vi "WinCI Convert Adv Options.vi"(4 "advanced options":variant) -> (1 "command options":u32)   [LabVIEW 2020, in "NI_SCC_WinCI.lvlib"]
uses:
  <vilib>/SourceControl/Providers/WinCI/NI_SCC_WinCI.lvlib
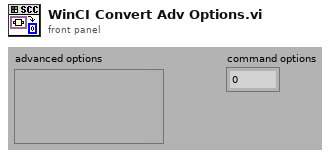
[diagram p1: front panel]
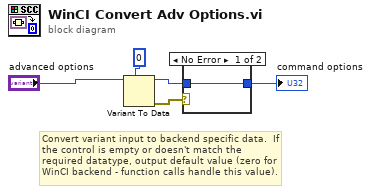
[diagram p0: block diagram]
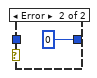
[diagram p2: hidden frame]
diagram:
  # "Convert variant input to backend specific data.  If the control is empty or doesn't match the required datatype, output default value (zero for WinCI backend - function calls handle this value)."
  n1 = Variant To Data(type=u32 0, Variant="advanced options") -> (data=w5:u32, error out=w4:errorcluster)  [unwired: 1 in]
  n2 = case shown="No Error" w4 {
    tunnel: [w6 u32 0] -> w1
    tunnel: w5 -> [w6 _]
    frame No Error {
    }
    frame Error {
    }
  }
  "command options" <- w1
